vi "DAQ IV bare.vi"() -> ()   [LabVIEW 2020]
panel:
  in  "End Current uA":dbl=2.0
  in  "Start Current uA":dbl=-2.0
  in  "Step uA":dbl=0.05
  in  "Delay Time s":dbl caption="Delay Time (s)"
  in  "AI channel":tag="Dev1/ai1"
  in  "AO channel":tag="Dev1/ao0"
  in  "samples per channel":i32=1000
  in  "base path":path=path "C:/Users/gyue/Box Sync/Guang Yue/data"
  in  "stop":bool
  in  "error in":T1
  out "error out":errorcluster
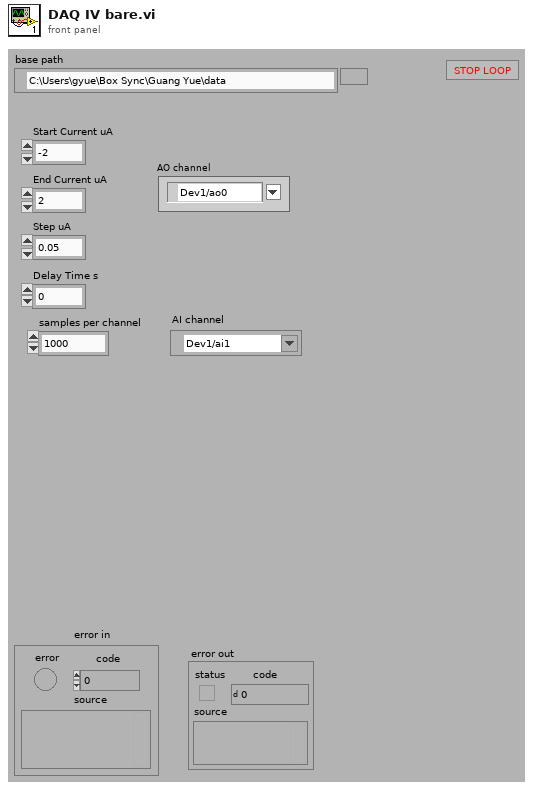
[diagram p1: front panel]
types:
  T1 = cluster{"error":bool, "code":i32, "source":string}
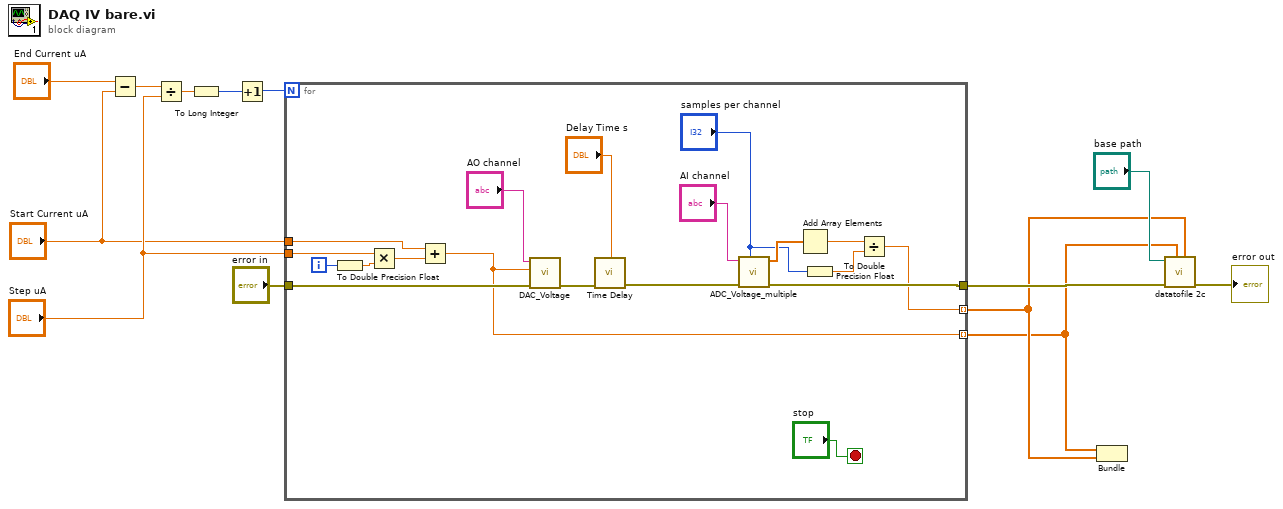
[diagram p0: block diagram]
diagram:
  n1 = Subtract(x="End Current uA", y="Start Current uA") -> (x-y=w14:dbl)
  n2 = Divide(x=w14, y="Step uA") -> (x/y=w13:dbl)
  n3 = To Long Integer(number=w13) -> (32bit integer=w7:i32)
  n4 = Increment(x=w7) -> (x+1=w12:i32)
  n5 = for {
    N: w12 -> [_]
    tunnel: [w27] -> w9
    tunnel: [w15] -> w1 mode=indexing
    tunnel: [w18] -> w3 mode=indexing
    tunnel: "error in" -> [w30]
    tunnel: "Step uA" -> [w25]
    tunnel: "Start Current uA" -> [w24]
    i -> [w33]
    stop <- "stop" stop-if-true
    n6 = To Double Precision Float(number=w33) -> (double precision float=w23:dbl)
    n7 = Multiply(x=w25, y=w23) -> (x*y=w32:dbl)
    n8 = Add(x=w24, y=w32) -> (x+y=w15:dbl)
    n9 = call "DAC_Voltage.vi"("error in"=w30, "Voltage"=w15, "Physical Channel(s)"="AO channel") -> ("error out"=w29:errorcluster)  [unwired: 8 in]
    n10 = call "Time Delay"("error in (no error)"=w29, "Delay Time (s)"="Delay Time s") -> ("error out"=w28:errorcluster)  [unwired: 9 in]
    n11 = call "ADC_Voltage_multiple.vi"("samples per channel"="samples per channel", "error in"=w28, "physical channels"="AI channel") -> ("error out"=w27:errorcluster, "data"=w22:dbl[])  [unwired: 7 in]
    n12 = Add Array Elements(numeric array=w22) -> (sum=w21:dbl)
    n13 = To Double Precision Float(number="samples per channel") -> (double precision float=w19:dbl)
    n14 = Divide(x=w21, y=w19) -> (x/y=w18:dbl)
  }
  n15 = Bundle(w1, w3) -> (w2:cluster{dbl[], dbl[]})  [unwired: 1 in]
  n16 = call "datatofile 2c.vi"("A2"=w3, "A1"=w1, "error in"=w9, "file path (dialog if empty)"="base path") -> ("error out"=→"error out":errorcluster)  [unwired: 7 in]
